vi "observacao_queued.vi"() -> ()   [LabVIEW 2012, in "Shared_160.lvlib"] (continued)
                n3063 = local read "MOV_IDX_DEC"() -> (w3919:bool)
                n3064 = global read "Global_Telescopio.vi" "CalLocal"() -> (w3926:bool)
                n3065 = global read "Global_Telescopio.vi" "CalGlobal"() -> (w3925:bool)
                n3066 = global read "Global_Telescopio.vi" "CoordDia"() -> (w3923:bool)
                n3067 = global read "Global_Telescopio.vi" "ObjCentrado"() -> (w3921:bool)
                n3068 = Build Array(w3926, w3925, w3924, w3923, w3922, w3921, w3920, w3919) -> (w3929:bool[])
                n3069 = Boolean Array To Number(Boolean array=w3929) -> (number=w3928:u32)
                n3070 = Number To Hexadecimal String(1:i16 2 ("width (-)"), 2:w3928) -> (0:w3918:string)
              }
              frame #1 {
                w3933 = "\t"
                # "Reseta Flag do comando oriundo\nda comunicação serial Aquisição"
                n3071 = local read "ChkPointPrecessed"() -> (w3930:bool)
                n3072 = local read "StrPointObjName"() -> (w3936:string)
                "NAME" <- w3936
                n3073 = local read "StrPointObjRA"() -> (w3935:string)
                "RA" <- w3935
                n3074 = local read "StrPointObjDEC"() -> (w3934:string)
                "DEC" <- w3934
                n3075 = case shown="True" w3930 {
                  tunnel: ["2000.0" ("Saída") w3940] -> w3931
                  frame False {
                  }
                  frame True {
                    n3076 = call "Calcula epoch.vi"() -> ("epoch"=w3943:dbl)  [unwired: 2 in]
                    n3077 = Number To Fractional String(number=w3943, precision (6)=i16 1) -> (F-format string=w3941:string)  [unwired: 2 in]
                    n3078 = call "Comma_to_Point.vi"("Lat_A"=w3941) -> ("Saída"=w3940:string)
                  }
                }
                n3079 = global write "Global_Telescopio.vi" "Centragem Via Aquisicao"(FALSE ("Centragem Via Aquisicao")) -> ()
                n3080 = local write "Processa Centragem"(TRUE) -> ()
                n3081 = global write "Global_Telescopio.vi" "NAME OBJETO"(w3936) -> ()
                n3082 = global write "Global_Telescopio.vi" "DEC AQUIS"(w3934) -> ()
                n3083 = global write "Global_Telescopio.vi" "RA AQUIS"(w3935) -> ()
                n3084 = Concatenate Strings(w3936, w3933, w3935, w3933, w3934) -> (w3932:string)
                n3085 = global write "Global_Telescopio.vi" "EPOCH AQUIS"(w3931) -> ()
              }
              frame #2 {
                w3944 = "\t"
                w3959 = FALSE ("use system decimal point (T)")
                w3960 = i16 1 ("precision (6)")
                n3086 = global read "Global_Telescopio.vi" "Right Ascention"() -> (w3950:string)
                n3087 = global read "Global_Telescopio.vi" "Calagem DEC"() -> (w3976:dbl)
                n3088 = global read "Global_Telescopio.vi" "Calagem AH"() -> (w3973:dbl)
                n3089 = global read "Global_Telescopio.vi" "Sideral Time"() -> (w3969:dbl)
                n3090 = global read "Global_Telescopio.vi" "Sideral time"() -> (w3947:string)
                n3091 = global read "Global_Telescopio.vi" "Hour Angle"() -> (w3948:string)
                n3092 = global read "Global_Telescopio.vi" "Declination"() -> (w3949:string)
                n3093 = global read "Global_Telescopio.vi" "TargetDEC"() -> (w3964:dbl)
                n3094 = local read "Offset DEC"() -> (w3962:dbl)
                n3095 = global read "Global_Telescopio.vi" "TargetRA"() -> (w3963:dbl)
                n3096 = local read "Offset RA"() -> (w3961:dbl)
                n3097 = global read "Global_Telescopio.vi" "PosDEC"() -> (w3967:dbl)
                n3098 = global read "Global_Telescopio.vi" "PosAH"() -> (w3970:dbl)
                n3099 = local read "UT"() -> (w3945:string)
                n3100 = Subtract(x=w3969, y=w3970) -> (x-y=w3968:dbl)
                n3101 = call "rad_hms.vi"("TRUE=HORA\nFALSE=GRAU"=TRUE ("TRUE=HORA\nFALSE=GRAU"), "Radiano"=w3963) -> ("Hora/Graus Texto Decimal"=w3957:string)  [unwired: 3 in]
                n3102 = call "rad_hms.vi"("TRUE=HORA\nFALSE=GRAU"=FALSE ("TRUE=HORA\nFALSE=GRAU"), "Radiano"=w3964) -> ("Hora/Graus Texto Decimal"=w3956:string)  [unwired: 3 in]
                n3103 = call "rad_hms.vi"("TRUE=HORA\nFALSE=GRAU"=TRUE ("TRUE=HORA\nFALSE=GRAU"), "Radiano"=w3968) -> ("Hora/Graus Texto Decimal"=w3955:string)  [unwired: 3 in]
                n3104 = call "rad_hms.vi"("TRUE=HORA\nFALSE=GRAU"=FALSE ("TRUE=HORA\nFALSE=GRAU"), "Radiano"=w3967) -> ("Hora/Graus Texto Decimal"=w3954:string)  [unwired: 3 in]
                n3105 = call "rad_hms.vi"("TRUE=HORA\nFALSE=GRAU"=TRUE, "Radiano"=w3973) -> ("Hora/Graus Texto Decimal"=w3953:string)  [unwired: 3 in]
                n3106 = call "rad_hms.vi"("TRUE=HORA\nFALSE=GRAU"=FALSE, "Radiano"=w3976) -> ("Hora/Graus Texto Decimal"=w3958:string)  [unwired: 3 in]
                n3107 = Number To Fractional String(use system decimal point (T)=w3959, number=w3962, precision (6)=w3960) -> (F-format string=w3952:string)  [unwired: 1 in]
                n3108 = Number To Fractional String(use system decimal point (T)=w3959, number=w3961, precision (6)=w3960) -> (F-format string=w3951:string)  [unwired: 1 in]
                n3109 = Concatenate Strings(w3957, w3944, w3956, w3944, w3955, w3944, w3954, w3944, w3953, w3944, w3958, w3944, w3952, w3944, w3951, w3944, w3950, w3944, w3949, w3944, w3948, w3944, w3947, w3944, w3945) -> (w3946:string)
              }
              frame #3 {
                w3982 = "\t"
                # "Condições atmosféricas"
                # "Dados de catálogo do Objeto"
                # "Tempo e posição do telescópio"
                # "Estados das variáveis de processos"
                n3110 = global read "Global_Telescopio.vi" "Data Arq LOG"() -> (w3997:string)
                n3111 = local read "AtmosferaStr"() -> (w3980:string)
                n3112 = Concatenate Strings("C:\\TCS\\LOG\\AP_" ("SOMENTE DIRETORIO"), w3997, ".TXT" ("SOMENTE DIRETORIO")) -> (w3996:string)
                n3113 = String To Path(string=w3996) -> (path=w3995:path)
                n3114 = call <vilib>:"Open_Create_Replace File.vi"("function (open:0)"=T9."open or create", "file path"=w3995) -> ("error out"=w3992:errorcluster, "refnum"=w3993:refnum<file>)  [unwired: 6 in, 2 out]
                n3115 = Concatenate Strings(w3985, w3982, w3984, w3982, w3980, w3982, w3983, "\r\n") -> (w3986:string)
                n3116 = Set File Position(refnum=w3993, from (0:start)=enum16{"start", "end", "current"}."end" ("pos mode (0:2)"), error in=w3992) -> (refnum out=w3979:refnum<file>, error out=w3978:errorcluster)  [unwired: 1 in]
                n3117 = Write to Binary File(file (use dialog)=w3979, data=w3986, error in=w3978, 5:FALSE ("prepend array or string size? (T)")) -> (refnum out=w3989:refnum<file>, error out=w3990:errorcluster)  [unwired: 2 in, 1 out]
                n3118 = Close File(refnum=w3989, error in=w3990) -> (error out=w3988:errorcluster)  [unwired: 1 out]
                n3119 = call <vilib>:"Simple Error Handler.vi"("error in (no error)"=w3988) -> ()  [unwired: 4 in, 5 out]
              }
            }
          }
        }
      }
      frame #4 {
        # "Abre Imagens"
        # "ABAS DE IMAGENS"
        n3120 = case shown="\"Image 1\", Default" "Tab Control" {
          frame "Image 1", Default {
            n3121 = disable-structure shown="Disabled" {
              frame Disabled {
                # "Imagem oriunda do\nconector BNC 1"
                n3122 = global read "Global_Telescopio.vi" "Tempo Atulização Cam 0"() -> (w4007:i16)
                n3123 = call "timepulse_Cam_0.vi"("de quantos segundos"=w4007) -> ("PULSO"=w4010:bool)  [unwired: 2 in]
                n3124 = Or(x="IMAGE 5", y=w4010) -> (x .or. y?=w4009:bool)
                n3125 = case shown="True" w4009 {
                  frame False {
                  }
                  frame True {
                    n3126 = call "AngeloRTV_Snap.vi"("PortNo"=u16 0) -> ("depth"=w4016:u8, "color table"=w4014:u32[], "rect"=w4017:T13, "flattened image data"=w4015:u8[])  [unwired: 2 in, 1 out]
                    n3127 = call <vilib>:"Draw Flattened Pixmap(6_1).vi"("bit depth(8)"=w4016, "rect"=w4017, "flattened pixmap data"=w4015, "color table"=w4014) -> ("new picture"=→"Image":picture)  [unwired: 5 in]
                    n3128 = call "Acerta_moldura.vi"("fator"=i16 1, "input cluster"=w4017) -> ("Draw Area Size"=w4011:cluster{"Width":u32, "Height":u32})  [unwired: 3 in]
                    n3129 = property on="Image" class="Pict"("Draw Area Size"=w4011) -> ()  [unwired: 2 in, 2 out]
                  }
                }
              }
              frame Enabled {
              }
            }
          }
          frame "All Sky" {
            n3130 = global read "Global_Telescopio.vi" "Tempo Atulização All Sky"() -> (w4019:i16)
            n3131 = call "timepulse_Cam_4.vi"("de quantos segundos"=w4019) -> ("PULSO"=w4020:bool)  [unwired: 2 in]
            n3132 = Or(x="IMAGE 2", y=w4020) -> (x .or. y?=w4021:bool)
            n3133 = case shown="True" w4021 {
              frame False {
              }
              frame True {
                n3134 = stacked-sequence {
                  frame #0 {
                    # "Deixado Propositalmente caso queira colocar uma camera no local do ALL SKY"
                    n3135 = case shown="True" "Case Constant\n(See Context Help) 16" {
                      frame False {
                      }
                      frame True {
                        # "Coloca a moldura na\nImagem"
                        # "Imagen da Cam Setada"
                        n3136 = call "AngeloRTV_Snap.vi"("PortNo"=u16 2) -> ("depth"=w4029:u8, "color table"=w4027:u32[], "rect"=w4030:T13, "flattened image data"=w4028:u8[])  [unwired: 2 in, 1 out]
                        n3137 = call "Acerta_moldura.vi"("fator"=i16 1, "input cluster"=w4030) -> ("Draw Area Size"=w4025:cluster{"Width":u32, "Height":u32})  [unwired: 3 in]
                        "Draw Area 2" <- w4025
                        n3138 = call <vilib>:"Draw Flattened Pixmap(6_1).vi"("bit depth(8)"=w4029, "rect"=w4030, "flattened pixmap data"=w4028, "color table"=w4027) -> ("new picture"=→"Image 2":picture)  [unwired: 5 in]
                        n3139 = property on="Image 2" class="Pict"("Draw Area Size"=w4025) -> ()  [unwired: 2 in, 2 out]
                      }
                    }
                  }
                  frame #1 {
                    # "Fora do ar\n12/02/2009"
                    n3140 = case shown="True" "Case Constant\n(See Context Help) 17" {
                      frame False {
                      }
                      frame True {
                        n3141 = stacked-sequence {
                          seq-local: [w4036 _] -> [_ w4045]
                          frame #0 {
                            n3142 = String To Path(string="C:\\TCSPD_TRABALHO\\IMAGE_TEMP.JPG") -> (path=w4040:path)
                            n3143 = call "URL Get HTTP Document.vi"("follow redirects (T)"="follow redirects (T)", "file path (NAP)"=w4040, "http URL"="http://200.131.64.207/allsky/imagens/allsky_opd.jpg") -> ("error out"=w4035:errorcluster, "file path out"=w4036:path, "header"=→"header":string)  [unwired: 1 in, 5 out]
                            "error out 2" <- w4035
                            n3144 = Unbundle By Name(w4035) -> ("status"=w4034:bool)
                            n3145 = case shown="True" w4034 {
                              frame False {
                              }
                              frame True {
                                n3146 = One Button Dialog(message="Erro durante a aquisição da Imagem do All Sky do site:\n\nhttp://200.131.64.207/allsky/imagens/allsky_opd.jpg") -> ()  [unwired: 1 in, 1 out]
                              }
                            }
                          }
                          frame #1 {
                            (unwired) path "\\\\200.131.64.207/allsky/imagens/allsky_opd.jpg\\" ("path to JPEG file")
                            (unwired) "\\Nasa - Earth From Outer Space.jpg" ("caminho final")
                            # "Isto não está sendo mais usado porémmantive se caso\nseja necessário a manipulação de arquivos com imagem"
                            # "fator de \nredução \nSomente\ninteiros até 6"
                            # "Sem nome de\narquivo ele abre\ncaixa de Diálogo"
                            # "Coloca a moldura na\nImagem"
                            # "Imagen da Cam Setada"
                            n3147 = call "Read JPEG File(6_1).vi"("path to JPEG file"=w4045) -> ("error out"=w4054:errorcluster, "flattened image data"=w4051:u8[], "rect"=w4050:T13, "colorTable"=w4053:u32[], "depth"=w4052:u8)  [unwired: 5 in, 1 out]
                            "error out 3" <- w4054
                            n3148 = String To Path(string="/root/Desktop/Simulador/Nasa - Earth From Outer Space.jpg" ("caminho final")) -> ()  [unwired: 1 out]
                            n3149 = call "Fator_Reducao.vi"("rect"=w4050, "flattened image in"=w4051, "Fator Tamanho"=i16 4) -> ("flattened image out"=w4049:u8[], "area figura x e y"=w4044:cluster{"X Resolution":i32, "Y Resolution":i32})  [unwired: 2 out]
                            n3150 = call "Webcam Flat to Picture.vi"("color table"=w4053, "depth 24/8"=w4052, "error in"=w4054, "rect in"=w4050, "flat image in"=w4049) -> ("error out"=→"error out 4":errorcluster, "picture"=w4043:picture)  [unwired: 2 in, 2 out]
                            n3151 = local write "Draw Area 2"(w4044) -> ()
                            n3152 = property on="Image 2" class="Pict"("Draw Area Size"=w4044) -> ()  [unwired: 2 in, 2 out]
                            n3153 = local write "Image 2"(w4043) -> ()
                            n3154 = call "Cria_path_local.vi"("caminho final"="\\allsky_opd.jpg") -> ()  [unwired: 3 in, 2 out]
                          }
                        }
                      }
                    }
                  }
                }
              }
            }
          }
          frame "Finder" {
            # "Imagem oriunda do\nconector BNC 4"
            n3155 = global read "Global_Telescopio.vi" "Tempo Atulização Cam 3"() -> (w4055:i16)
            n3156 = call "timepulse_Cam_3.vi"("de quantos segundos"=w4055) -> ("PULSO"=w4056:bool)  [unwired: 2 in]
            n3157 = Or(x="IMAGE 4", y=w4056) -> (x .or. y?=w4058:bool)
            n3158 = case shown="True" w4058 {
              frame False {
              }
              frame True {
                n3159 = stacked-sequence {
                  frame #0 {
                    n3160 = call "AngeloRTV_Snap.vi"("PortNo"=u16 3) -> ("depth"=w4064:u8, "color table"=w4062:u32[], "rect"=w4065:T13, "flattened image data"=w4063:u8[])  [unwired: 2 in, 1 out]
                    n3161 = call "Acerta_moldura.vi"("fator"=i16 1, "input cluster"=w4065) -> ("Draw Area Size"=w4059:cluster{"Width":u32, "Height":u32})  [unwired: 3 in]
                    "Draw Area 4" <- w4059
                    n3162 = call <vilib>:"Draw Flattened Pixmap(6_1).vi"("bit depth(8)"=w4064, "rect"=w4065, "flattened pixmap data"=w4063, "color table"=w4062) -> ("new picture"=→"Image 4":picture)  [unwired: 5 in]
                    n3163 = property on="Image 4" class="Pict"("Draw Area Size"=w4059) -> ()  [unwired: 2 in, 2 out]
                  }
                  frame #1 {
                    n3164 = case shown="True" "Case Constant\n(See Context Help) 18" {
                      frame False {
                      }
                      frame True {
                        # "Isto não está sendo mais usado porémmantive se caso\nseja necessário a manipulação de arquivos com imagem"
                        # "fator de \nredução \nSomente\ninteiros até 6"
                        # "Sem nome de\narquivo ele abre\ncaixa de Diálogo"
                        # "Coloca a moldura na\nImagem"
                        # "Imagen da Cam Setada"
                        n3165 = call "Cria_path_local.vi"("caminho final"="\\Nasa - Earth From Outer Space.jpg") -> ("Saida Path inteiro"=w4070:path)  [unwired: 3 in, 1 out]
                        n3166 = call "Read JPEG File(6_1).vi"("path to JPEG file"=w4070) -> ("error out"=w4079:errorcluster, "flattened image data"=w4076:u8[], "rect"=w4075:T13, "colorTable"=w4078:u32[], "depth"=w4077:u8)  [unwired: 5 in, 1 out]
                        n3167 = String To Path(string="/root/Desktop/Simulador/Nasa - Earth From Outer Space.jpg" ("caminho final")) -> ()  [unwired: 1 out]
                        n3168 = call "Fator_Reducao.vi"("rect"=w4075, "flattened image in"=w4076, "Fator Tamanho"=i16 1) -> ("flattened image out"=w4074:u8[], "area figura x e y"=w4068:cluster{"X Resolution":i32, "Y Resolution":i32})  [unwired: 2 out]
                        n3169 = local write "Draw Area 4"(w4068) -> ()
                        n3170 = property on="Image 4" class="Pict"("Draw Area Size"=w4068) -> ()  [unwired: 2 in, 2 out]
                        n3171 = call "Webcam Flat to Picture.vi"("color table"=w4078, "depth 24/8"=w4077, "error in"=w4079, "rect in"=w4075, "flat image in"=w4074) -> ("picture"=w4069:picture)  [unwired: 2 in, 3 out]
                        n3172 = local write "Image 4"(w4069) -> ()
                      }
                    }
                  }
                }
              }
            }
          }
          frame "Telescope" {
            # "Imagem oriunda do\nconector BNC 2"
            n3173 = global read "Global_Telescopio.vi" "Tempo Atulização Cam 1"() -> (w4080:i16)
            n3174 = call "timepulse_Cam_1.vi"("de quantos segundos"=w4080) -> ("PULSO"=w4081:bool)  [unwired: 2 in]
            n3175 = Or(x="IMAGE 3", y=w4081) -> (x .or. y?=w4082:bool)
            n3176 = case shown="True" w4082 {
              frame False {
              }
              frame True {
                n3177 = case shown="True" "Case Constant\n(See Context Help) 19" {
                  frame False {
                  }
                  frame True {
                    n3178 = call "AngeloRTV_Snap.vi"("PortNo"=u16 1) -> ("depth"=w4090:u8, "color table"=w4088:u32[], "rect"=w4091:T13, "flattened image data"=w4089:u8[])  [unwired: 2 in, 1 out]
                    n3179 = call <vilib>:"Draw Flattened Pixmap(6_1).vi"("bit depth(8)"=w4090, "rect"=w4091, "flattened pixmap data"=w4089, "color table"=w4088) -> ("new picture"=→"Image 3":picture)  [unwired: 5 in]
                    n3180 = call "Acerta_moldura.vi"("fator"=i16 1, "input cluster"=w4091) -> ("Draw Area Size"=w4085:cluster{"Width":u32, "Height":u32})  [unwired: 3 in]
                    "Draw Area 3" <- w4085
                    n3181 = property on="Image 3" class="Pict"("Draw Area Size"=w4085) -> ()  [unwired: 2 in, 2 out]
                  }
                }
              }
            }
          }
          frame "Image 3" {
            # "Imagem oriunda do\nconector BNC 3"
            n3182 = global read "Global_Telescopio.vi" "Tempo Atulização Cam 2"() -> (w4093:i16)
            n3183 = call "timepulse_Cam_2.vi"("de quantos segundos"=w4093) -> ("PULSO"=w4094:bool)  [unwired: 2 in]
            n3184 = Or(x="IMAGE 6", y=w4094) -> (x .or. y?=w4096:bool)
            n3185 = case shown="True" w4096 {
              frame False {
              }
              frame True {
                n3186 = call "AngeloRTV_Snap.vi"("PortNo"=u16 2) -> ("depth"=w4102:u8, "color table"=w4100:u32[], "rect"=w4103:T13, "flattened image data"=w4101:u8[])  [unwired: 2 in, 1 out]
                n3187 = call "Acerta_moldura.vi"("fator"=i16 1, "input cluster"=w4103) -> ("Draw Area Size"=w4097:cluster{"Width":u32, "Height":u32})  [unwired: 3 in]
                n3188 = call <vilib>:"Draw Flattened Pixmap(6_1).vi"("bit depth(8)"=w4102, "rect"=w4103, "flattened pixmap data"=w4101, "color table"=w4100) -> ("new picture"=→"Image 3a":picture)  [unwired: 5 in]
                n3189 = property on="Image 3a" class="Pict"("Draw Area Size"=w4097) -> ()  [unwired: 2 in, 2 out]
              }
            }
          }
          frame "Test Only" {
          }
        }
        n3190 = global read "Global_Telescopio.vi" "Caminho camera"() -> (w4004:string)
        n3191 = global read "Global_Telescopio.vi" "stop"() -> (w4005:bool)
        n3192 = call "Greatek.vi"("error in (no error)"="error in (no error)", "Boolean"=w4005, "name or relative path"=w4004, ".NET Refnum in"="PictureBox") -> ("error out"=→"error out 5":errorcluster)  [unwired: 7 in]
      }
      frame #5 {
        w4108 = u16 3 items=["Alarme", "Atencao", "Erro", "Ocupado", "TBD", "LCB", "Trapeira", "Paravento", "DomoRap", "DomoCW", "DomoCCW", "TBD", "Em movimento", "TBD"] ("NomeStatus")
        # "JANELA DE STATUS"
        n3193 = local read "ChkDomeEnable"() -> (w4119:bool)
        n3194 = local read "Flag Stop"() -> (w4114:bool)
        n3195 = case shown="True" w4119 {
          tunnel: [TRUE ("AUX LAMPADA") w4273] -> w4118
          frame False {
          }
          frame True {
            w4279 = u16 3 items=["Alarme", "Atencao", "Erro", "Ocupado", "TBD", "LCB", "Trapeira", "Paravento", "DomoRap", "DomoCW", "DomoCCW", "TBD", "Em movimento", "TBD"] ("NomeStatus")
            n3196 = local read "Dome on Target"() -> (w4276:bool)
            n3197 = local read "statCUP"() -> (w4278:i32)
            n3198 = call "Bit Status CUP.vi"("NomeStatus"=w4279) -> ("StatBit"=w4275:bool)
            n3199 = Equal To 0?(x=w4278) -> (x = 0?=w4277:bool)
            n3200 = Not(x=w4275) -> (.not. x?=w4274:bool)
            n3201 = Compound Arithmetic op=AND(w4277, w4276, w4274) -> (w4273:bool)
          }
        }
        n3202 = case shown="True" w4114 {
          tunnel: [FALSE w4266] -> w4113
          frame False {
          }
          frame True {
            w4270 = u16 3 items=["Alarme", "Atencao", "Erro", "Ocupado", "TBD", "LCB", "Trapeira", "Paravento", "DomoRap", "DomoCW", "DomoCCW", "TBD", "Em movimento", "TBD"] ("NomeStatus")
            n3203 = local read "statCUP"() -> (w4269:i32)
            n3204 = call "Bit Status CUP.vi"("NomeStatus"=w4270) -> ("StatBit"=w4271:bool)
            n3205 = Equal To 0?(x=w4269) -> (x = 0?=w4268:bool)
            n3206 = Not(x=w4271) -> (.not. x?=w4267:bool)
            n3207 = Compound Arithmetic op=AND(w4268, w4267) -> (w4266:bool)
          }
        }
        n3208 = local read "Apontou"() -> (w4126:bool)
        n3209 = local read "BtUtilZenith"() -> (w4134:bool)
        n3210 = local read "BtUtilPark"() -> (w4133:bool)
        n3211 = local read "BtUtilZenith"() -> (w4132:bool)
        n3212 = local read "ECASS"() -> (w4131:bool)
        n3213 = local read "FLAT-FIELD"() -> (w4130:bool)
        n3214 = local read "Flag de erro p/ apagar lampada"() -> (w4109:bool)
        n3215 = call "Bit Status CUP.vi"("NomeStatus"=w4108) -> ("StatBit"=w4107:bool)
        n3216 = Not(x=w4107) -> (.not. x?=w4106:bool)
        n3217 = local read "DEC on Target"() -> (w4120:bool)
        n3218 = local read "RA on Target"() -> (w4121:bool)
        n3219 = Compound Arithmetic op=OR(w4126, w4134, w4133, w4132, w4131, w4130) -> (w4127:bool)
        n3220 = And(x=w4127, y="AUX ABA") -> (x .and. y?=w4129:bool)
        n3221 = Compound Arithmetic op=AND(w4109, w4106) -> (w4105:bool)
        n3222 = case shown="False" w4127 {
          selector: w4127 -> [w4287 _]
          frame False {
            n3223 = Not(x=w4287) -> (.not. x?=w4288:bool)
            n3224 = local write "AUX ABA"(w4288) -> ()
          }
          frame True {
          }
        }
        n3225 = Not(x=w4121) -> (.not. x?=w4122:bool)
        n3226 = Not(x=w4120) -> (.not. x?=w4124:bool)
        n3227 = Not(x=w4118) -> (.not. x?=w4123:bool)
        n3228 = Compound Arithmetic op=AND(w4121, w4120, w4118) -> (w4117:bool)
        n3229 = case shown="True" w4129 {
          selector: w4129 -> [_ w4291]
          frame False {
          }
          frame True {
            # "Liga a câmera de monitoramento"
            # "Ligar a lâmpada pra a câmera"
            n3230 = Not(x=w4291) -> (.not. x?=w4290:bool)
            n3231 = local write "AUX ABA"(w4290) -> ()
            n3232 = local write "Apontou"(w4290) -> ()
            n3233 = local write "AUX LAMPADA"(TRUE ("AUX LAMPADA")) -> ()
            n3234 = local write "Tab Control"(T1."Image 1" ("Tab Control")) -> ()
          }
        }
        n3235 = Compound Arithmetic op=OR(w4122, w4124, w4123) -> (w4125:bool)
        n3236 = And(x=w4117, y="AUX LAMPADA") -> (x .and. y?=w4115:bool)
        n3237 = Or(x=w4115, y=w4113) -> (x .or. y?=w4110:bool)
        n3238 = Or(x=w4110, y=w4105) -> (x .or. y?=w4111:bool)
        n3239 = case shown="True" w4125 {
          selector: w4125 -> [_ w4286]
          frame False {
          }
          frame True {
            n3240 = local write "AUX LAMPADA"(w4286) -> ()
          }
        }
        n3241 = case shown="True" w4111 {
          selector: w4111 -> [_ w4284]
          frame False {
          }
          frame True {
            w4281 = u16 4 items=["ZERO", "AH", "DEC", "TUBO", "CUP"] ("Controlador")
            n3242 = Not(x=w4284) -> (.not. x?=w4280:bool)
            n3243 = local write "AUX LAMPADA"(w4280) -> ()
            n3244 = local write "Flag Stop"(w4280) -> ()
            n3245 = local write "Flag de erro p/ apagar lampada"(w4280) -> ()
            n3246 = local write "Tab Control"(T1."Test Only" ("Tab Control")) -> ()
            n3247 = call "Monta Comando.vi"("Comando"="DESLIGAR", "Dispositivo"="LAMP_CAM", "Controlador"=w4281) -> ()  [unwired: 4 in, 3 out]
          }
        }
        n3248 = global read "Global_Telescopio.vi" "Enable ventilador"() -> (w4112:bool)
        n3249 = Tick Count (ms)() -> (millisecond timer value=w4137:u32)
        n3250 = Subtract(x=w4137, y=w4136) -> (x-y=→"dt":u32)
        n3251 = case shown="True" w4112 {
          frame False {
          }
          frame True {
            w4143 = u16 3 items=["Alarme", "Atencao", "Erro", "Ocupado", "TBD", "LCB", "Trapeira", "Paravento", "DomoRap", "DomoCW", "DomoCCW", "TBD", "Em movimento", "TBD"] ("NomeStatus")
            n3252 = global read "Global_Telescopio.vi" "Hora vent inicial"() -> (w4140:string)
            n3253 = global read "Global_Telescopio.vi" "Hora vent final"() -> (w4139:string)
            n3254 = call "Bit Status TUBO.vi"("NomeStatus"=w4143) -> ("StatBit"=w4142:bool)
            n3255 = call "Comp-HorarioSeg.vi"("Lower limit"=w4140, "Upper limit"=w4139) -> ("In Range?"=w4138:bool)
            n3256 = Not(x=w4142) -> (.not. x?=w4141:bool)
            n3257 = case shown="\"erro_desligar\"" "xxz" {
              tunnel: [w4146 w4170 w4195 w4199 w4212 w4218 w4231] -> w4144
              tunnel: w4138 -> [_ _ w4194 _ w4214 _ w4232]
              tunnel: w4141 -> [w4147 w4171 _ w4198 w4213 w4217 _]
              frame "erro_ligar" {
                n3258 = case shown="True" w4147 {
                  tunnel: ["erro_ligar" w4149] -> w4146
                  frame False {
                  }
                  frame True {
                    w4158 = u16 3 items=["ZERO", "AH", "DEC", "TUBO", "CUP"] ("Controlador")
                    # "super erro"
                    n3259 = call "Monta Comando.vi"("Comando"="LIGAR", "Dispositivo"="VENTILADOR", "Controlador"=w4158) -> ("Resposta"=w4161:string)  [unwired: 4 in, 2 out]
                    n3260 = String Subset(string=w4161, length (rest)=3 ("length (rest)")) -> (substring=w4155:string)  [unwired: 1 in]
                    n3261 = Equal?(x=w4155, y="ACK") -> (x = y?=w4151:bool)
                    n3262 = case shown="False" w4151 {
                      tunnel: [w4162 FALSE] -> w4152
                      tunnel: "erro_ligar" -> [w4163 _]
                      tunnel: [w4163 "espera_desligar"] -> w4150
                      frame False {
                        n3263 = Increment(x="erro lig") -> (x+1=w4164:i32)
                        n3264 = local write "erro lig"(w4164) -> ()
                        n3265 = Greater Or Equal?(x=w4164, y=3) -> (x >= y?=w4162:bool)
                        n3266 = case shown="True" w4162 {
                          frame False {
                          }
                          frame True {
                            w4167 = "Erro de acionamento do ventilador do tubo" ("SYSTEM MESSAGES")
                            n3267 = call "Monta_Mensagem.vi"("Mensagem"=w4167) -> ()  [unwired: 2 in]
                            n3268 = call "Salva_systems_messages.vi"("Mensagem"=w4167) -> ()  [unwired: 5 in]
                          }
                        }
                      }
                      frame True {
                      }
                    }
                    n3269 = Select(t="espera_desligar", s=w4152, f=w4150) -> (s? t:f=w4149:string)
                  }
                }
              }
              frame "erro_desligar" {
                n3270 = case shown="True" w4171 {
                  tunnel: ["erro_desligar" w4173] -> w4170
                  frame False {
                  }
                  frame True {
                    w4183 = u16 3 items=["ZERO", "AH", "DEC", "TUBO", "CUP"] ("Controlador")
                    # "super erro"
                    n3271 = call "Monta Comando.vi"("Comando"="DESLIGAR", "Dispositivo"="VENTILADOR", "Controlador"=w4183) -> ("Resposta"=w4181:string)  [unwired: 4 in, 2 out]
                    n3272 = String Subset(string=w4181, length (rest)=3 ("length (rest)")) -> (substring=w4179:string)  [unwired: 1 in]
                    n3273 = Equal?(x=w4179, y="ACK") -> (x = y?=w4178:bool)
                    n3274 = case shown="False" w4178 {
                      tunnel: [w4186 FALSE] -> w4177
                      tunnel: "erro_desligar" -> [w4187 _]
                      tunnel: [w4187 "aguardando _ligar"] -> w4175
                      frame False {
                        n3275 = Increment(x="erro des") -> (x+1=w4189:i32)
                        n3276 = local write "erro des"(w4189) -> ()
                        n3277 = Greater Or Equal?(x=w4189, y=3) -> (x >= y?=w4186:bool)
                        n3278 = case shown="True" w4186 {
                          frame False {
                          }
                          frame True {
                            w4191 = "Erro de acionamento do ventilador do tubo" ("SYSTEM MESSAGES")
                            n3279 = call "Monta_Mensagem.vi"("Mensagem"=w4191) -> ()  [unwired: 2 in]
                            n3280 = call "Salva_systems_messages.vi"("Mensagem"=w4191) -> ()  [unwired: 5 in]
                          }
                        }
                      }
                      frame True {
                      }
                    }
                    n3281 = Select(t="aguardando _ligar", s=w4177, f=w4175) -> (s? t:f=w4173:string)
                  }
                }
              }
              frame "inicio", Default {
                n3282 = Select(t="ligar", s=w4194, f="desligar") -> (s? t:f=w4195:string)
              }
              frame "ligar" {
                n3283 = case shown="True" w4198 {
                  tunnel: ["ligar" w4202] -> w4199
                  frame False {
                  }
                  frame True {
                    w4209 = u16 3 items=["ZERO", "AH", "DEC", "TUBO", "CUP"] ("Controlador")
                    n3284 = call "Monta Comando.vi"("Comando"="LIGAR", "Dispositivo"="VENTILADOR", "Controlador"=w4209) -> ("Resposta"=w4207:string)  [unwired: 4 in, 2 out]
                    n3285 = String Subset(string=w4207, length (rest)=3 ("length (rest)")) -> (substring=w4205:string)  [unwired: 1 in]
                    n3286 = Equal?(x=w4205, y="ACK") -> (x = y?=w4201:bool)
                    n3287 = Select(t="espera_desligar", s=w4201, f="erro_ligar") -> (s? t:f=w4202:string)
                  }
                }
              }
              frame "espera_desligar" {
                n3288 = case shown="False" w4214 {
                  tunnel: w4213 -> [_ _]
                  tunnel: ["desligar" "espera_desligar"] -> w4212
                  frame False {
                    # "Já ligou mas saiu da faixa e deve desligar"
                  }
                  frame True {
                    # "Já ligou mas está na faixa"
                  }
                }
              }
              frame "desligar" {
                n3289 = case shown="True" w4217 {
                  tunnel: ["desligar" w4220] -> w4218
                  frame False {
                  }
                  frame True {
                    w4228 = u16 3 items=["ZERO", "AH", "DEC", "TUBO", "CUP"] ("Controlador")
                    n3290 = call "Monta Comando.vi"("Comando"="DESLIGAR", "Dispositivo"="VENTILADOR", "Controlador"=w4228) -> ("Resposta"=w4226:string)  [unwired: 4 in, 2 out]
                    n3291 = String Subset(string=w4226, length (rest)=3 ("length (rest)")) -> (substring=w4224:string)  [unwired: 1 in]
                    n3292 = Equal?(x=w4224, y="ACK") -> (x = y?=w4223:bool)
                    n3293 = Select(t="aguardando _ligar", s=w4223, f="erro_desligar") -> (s? t:f=w4220:string)
                  }
                }
              }
              frame "aguardando _ligar" {
                n3294 = case shown="True" w4232 {
                  tunnel: ["aguardando _ligar" "ligar"] -> w4231
                  frame False {
                  }
                  frame True {
                  }
                }
              }
            }
            n3295 = local write "xxz"(w4144) -> ()
          }
        }
        n3296 = stacked-sequence {
          frame #0 {
            n3297 = Get Date/Time String(want seconds? (F)=TRUE ("Boolean")) -> (time string=w4237:string)  [unwired: 2 in, 1 out]
            n3298 = In Range and Coerce(upper limit="16:00:01", x=w4237, lower limit="15:59:59" ("upper limit")) -> (In Range?=w4236:bool)  [unwired: 1 out]
            n3299 = In Range and Coerce(upper limit="17:45:01", x=w4237, lower limit="17:44:59" ("upper limit")) -> (In Range?=w4235:bool)  [unwired: 1 out]
            n3300 = case shown="True" w4235 {
              selector: w4235 -> [_ w4243]
              frame False {
              }
              frame True {
                "Flag desligar" <- w4243
              }
            }
            n3301 = case shown="True" w4236 {
              selector: w4236 -> [_ w4244]
              frame False {
              }
              frame True {
                "Flag ligar" <- w4244
              }
            }
          }
          frame #1 {
            n3302 = local read "Flag ligar"() -> (w4246:bool)
            n3303 = local read "Flag desligar"() -> (w4245:bool)
            n3304 = Or(x=w4246, y=w4245) -> (x .or. y?=w4247:bool)
            n3305 = case shown="True" w4247 {
              tunnel: w4246 -> [_ w4248]
              tunnel: w4245 -> [_ w4250]
              frame False {
              }
              frame True {
                w4254 = u16 3 items=["Alarme", "Atencao", "Erro", "Ocupado", "TBD", "LCB", "Trapeira", "Paravento", "DomoRap", "DomoCW", "DomoCCW", "TBD", "Em movimento", "TBD"] ("NomeStatus")
                n3306 = call "Bit Status TUBO.vi"("NomeStatus"=w4254) -> ("StatBit"=w4253:bool)
                n3307 = Not(x=w4253) -> (.not. x?=w4249:bool)
                n3308 = And(x=w4249, y=w4250) -> (x .and. y?=w4251:bool)
                n3309 = And(x=w4248, y=w4249) -> (x .and. y?=w4252:bool)
                n3310 = case shown="True" w4251 {
                  selector: w4251 -> [_ w4259]
                  frame False {
                  }
                  frame True {
                    w4255 = u16 3 items=["ZERO", "AH", "DEC", "TUBO", "CUP"] ("Controlador")
                    n3311 = Not(x=w4259) -> (.not. x?=w4258:bool)
                    n3312 = local write "Flag desligar"(w4258) -> ()
                    n3313 = call "Monta Comando.vi"("Comando"="DESLIGAR", "Dispositivo"="VENTILADOR", "Controlador"=w4255) -> ()  [unwired: 4 in, 3 out]
                  }
                }
                n3314 = case shown="True" w4252 {
                  selector: w4252 -> [_ w4264]
                  frame False {
                  }
                  frame True {
                    w4262 = u16 3 items=["ZERO", "AH", "DEC", "TUBO", "CUP"] ("Controlador")
                    n3315 = Not(x=w4264) -> (.not. x?=w4263:bool)
                    n3316 = local write "Flag ligar"(w4263) -> ()
                    n3317 = call "Monta Comando.vi"("Comando"="LIGAR", "Dispositivo"="VENTILADOR", "Controlador"=w4262) -> ()  [unwired: 4 in, 3 out]
                  }
                }
              }
            }
          }
        }
      }
    }
    n3318 = Wait Until Next ms Multiple(millisecond multiple=u32 100) -> ()  [unwired: 1 out]
    n3319 = global read "Global_Telescopio.vi" "stop"() -> (w75:bool)
    n3320 = Or(x=w75, y="sair") -> (x .or. y?=w76:bool)
  }
  n3321 = local write "ChkDomeEnable"(TRUE ("ChkDomeEnable")) -> ()
  n3322 = global write "Global_Telescopio.vi" "Default Met"(FALSE ("ChkDomeEnable")) -> ()
  n3323 = Get Date/Time In Seconds() -> (seconds since 1Jan1904=→"alarm Time":timestamp)
  n3324 = property on="Mensage Alarme" class="Str"("Visible"=w17, "Blinking"=TRUE) -> ()  [unwired: 2 in, 2 out]
  n3325 = property on="Setup, Pointing & Guiding" class="TabCtl (strict)"("MultColors"=TRUE ("Allow Multiple Colors")) -> ()  [unwired: 2 in, 2 out]
  n3326 = flat-sequence {
    tunnel: w1 -> [_]
    frame #0 {
      # "Comando EXIT\nP/ O VI QBRIDGE"
      # "Libera as filas do focalizador"
      n3327 = global read "Global_Telescopio.vi" "queueSUB"() -> (w4296:refnum<queue>)
      n3328 = global read "Global_Telescopio.vi" "queuePUSH"() -> (w4295:refnum<queue>)
      n3329 = Enqueue Element(queue=w4295, element="AbortBridge") -> (queue out=w4294:refnum<queue>)  [unwired: 2 in, 2 out]
      n3330 = Release Queue(queue=w4296) -> ()  [unwired: 2 in, 3 out]
      n3331 = Release Queue(queue=w4294) -> ()  [unwired: 2 in, 3 out]
    }
  }
  n3332 = case shown="True" FALSE {
    tunnel: w1 -> [_ w4297]
    frame False {
    }
    frame True {
      n3333 = Quit LabVIEW(quit? (T)=w4297) -> ()
    }
  }
  "Flag Alarm" <- w17
  "shutterTimeOld" <- 0 ("shutterTimeOld")
  "sendCommandShutter" <- FALSE ("writeShutterLog")
  "timeStatShutterAlert" <- 0 ("timeStatShutterAlert")
